vi "Sweep 2.0 Tester.vi"() -> ()   [LabVIEW 2013]
panel:
  out "Waveform Chart Time":dbl(graph)
  out "Waveform Chart Centers":i32(graph)
  out "Loop Counter":i32
  in  "Stop Button":bool
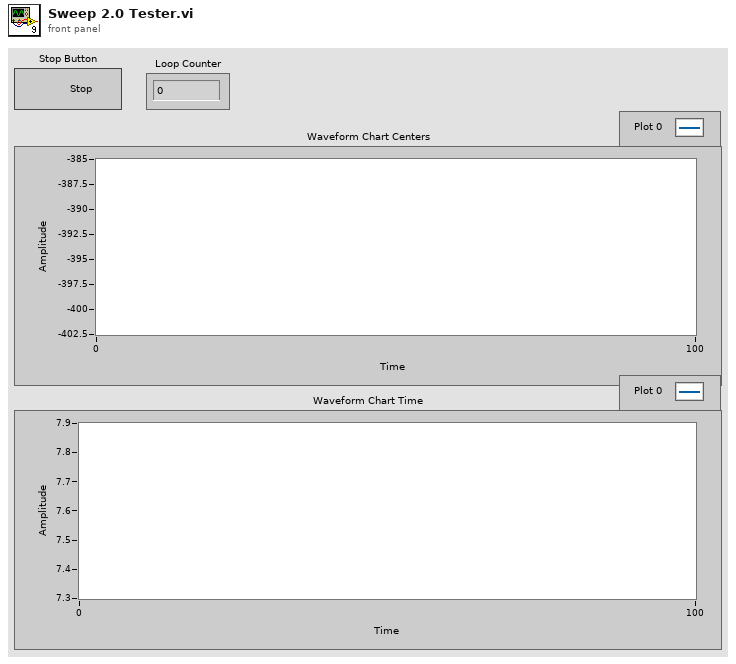
[diagram p1: front panel]
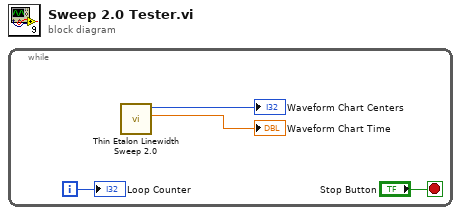
[diagram p0: block diagram]
diagram:
  n1 = while {
    i -> [w3]
    stop <- "Stop Button" stop-if-true
    n2 = call "Thin Etalon Linewidth Sweep 2.0.vi"() -> ("Time Elapsed"=→"Waveform Chart Time":dbl, "Center Position"=→"Waveform Chart Centers":i32)  [unwired: 6 in, 4 out]
    "Loop Counter" <- w3
  }
